vi "Set Image.vi"(8 "error in (no error)":errorcluster, 11 "CCDCamera in":refnum<class "CCDCamera.lvclass">) -> (0 "error out":errorcluster, 3 "CCDCamera out":refnum<class "CCDCamera.lvclass">)   [LabVIEW 2018, in "CCDCamera.lvclass"]
uses:
  CCDCamera.lvclass
  CCDCamera.lvclass/CCDCamera.ctl
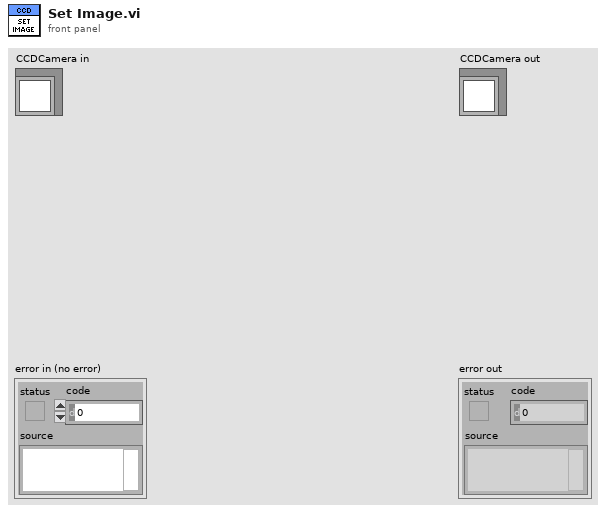
[diagram p1: front panel]
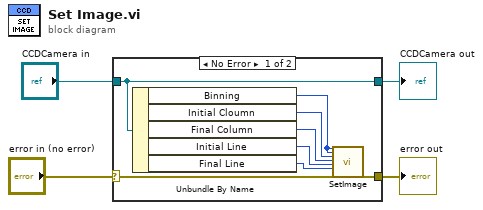
[diagram p0: block diagram]
diagram:
  n1 = case shown="No Error" "error in (no error)" {
    selector: "error in (no error)" -> [w11 w14]
    tunnel: [w12 w14] -> w3
    tunnel: [w10 w13] -> w1
    tunnel: "CCDCamera in" -> [w10 w13]
    frame No Error {
      n2 = Unbundle By Name(w10) -> ("Binning"=w9:u16, "Initial Cloumn"=w8:u16, "Final Column"=w7:u16, "Initial Line"=w6:u16, "Final Line"=w5:u16)
      n3 = call <userlib>:"SetImage.vi"("hbin"=w9, "vbin"=w9, "hstart"=w8, "hend"=w7, "vstart"=w6, "vend"=w5, "error in (no error)"=w11) -> ("error out"=w12:errorcluster)  [unwired: 19 in, 1 out]
    }
    frame Error {
    }
  }
  "error out" <- w3
  "CCDCamera out" <- w1
